vi "Second_max.vi"(11 "Array":dbl[](array[numeric])) -> (3 "AP3":dbl)   [LabVIEW 2022 SP3]
uses:
  5a59ef4f-e42f-4e8e-a549-f7ff9033d643.vi
  <vilib>/Comparison/Less/Less Functor/Less Functor.lvclass
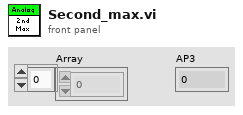
[diagram p1: front panel]
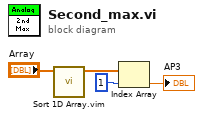
[diagram p0: block diagram]
diagram:
  n1 = call "Sort 1D Array.vim"("unsorted array"="Array") -> ("sorted array"=w2:dbl[])  [unwired: 10 in]
  n2 = Index Array(array=w2, index=1) -> (element=→"AP3":dbl)
